vi "LAS-CTS_NDFilterScanCharge.vi"() -> ()   [LabVIEW 2024]
uses:
  <vilib>/httpClient/LabVIEWHTTPClient.lvlib
  <vilib>/Analysis/NI_AALBase.lvlib
panel:
  out "Ion Charge Chart":dbl(graph)
  out "Ion Charge (pC)":dbl format="%.3g"
  in  "Keithly":refnum<visa-resource-name>
  out "Laser Energy Chart":dbl(graph)
  out "Average Laser Energy (uJ)":dbl format="%.3g"
  out "ND Filter Position":i32
  in  "file path (use dialog)":path
  in  "# of Positions":i32
  in  "Step Size":i32
  in  "ND Filter":refnum<visa-resource-name>
  in  "Number of Pulses":i32
  out "number of measurements":i32
  out "Laser Energy (uJ)":dbl
  in  "Energy Meter":refnum<visa-resource-name>
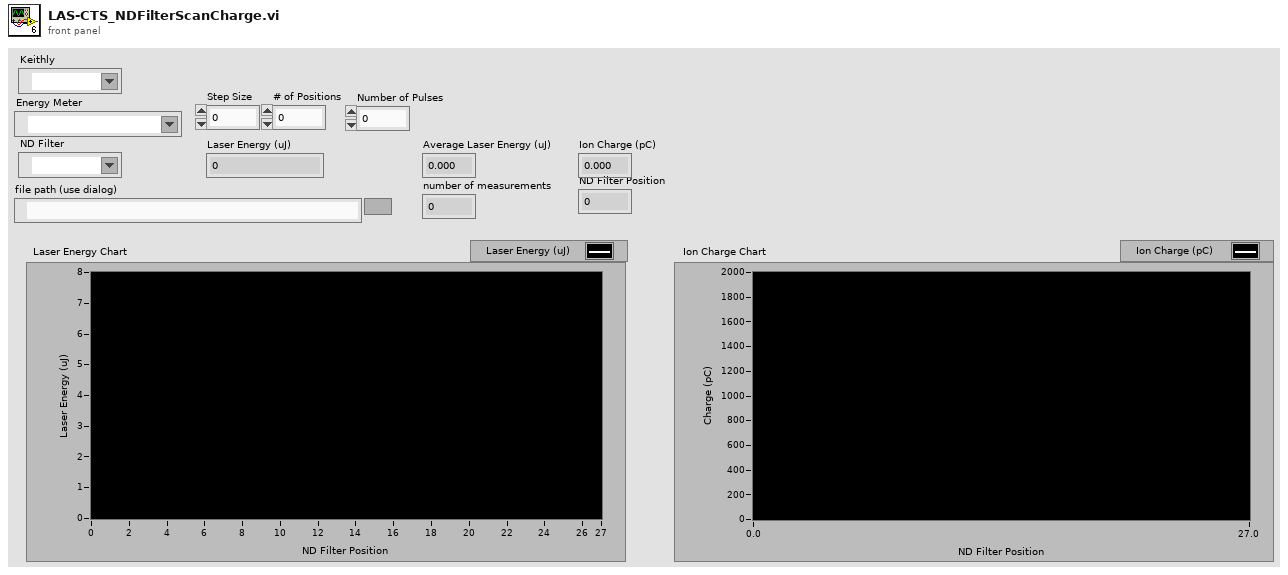
[diagram p1: front panel]
types:
  T1 = enum16{"open", "replace", "create", "open or create", "replace or create", "replace or create with confirmation"}
  T2 = typedef "LabVIEWHTTPClient.lvlib/ClientHandle.ctl" = refnum<k1>
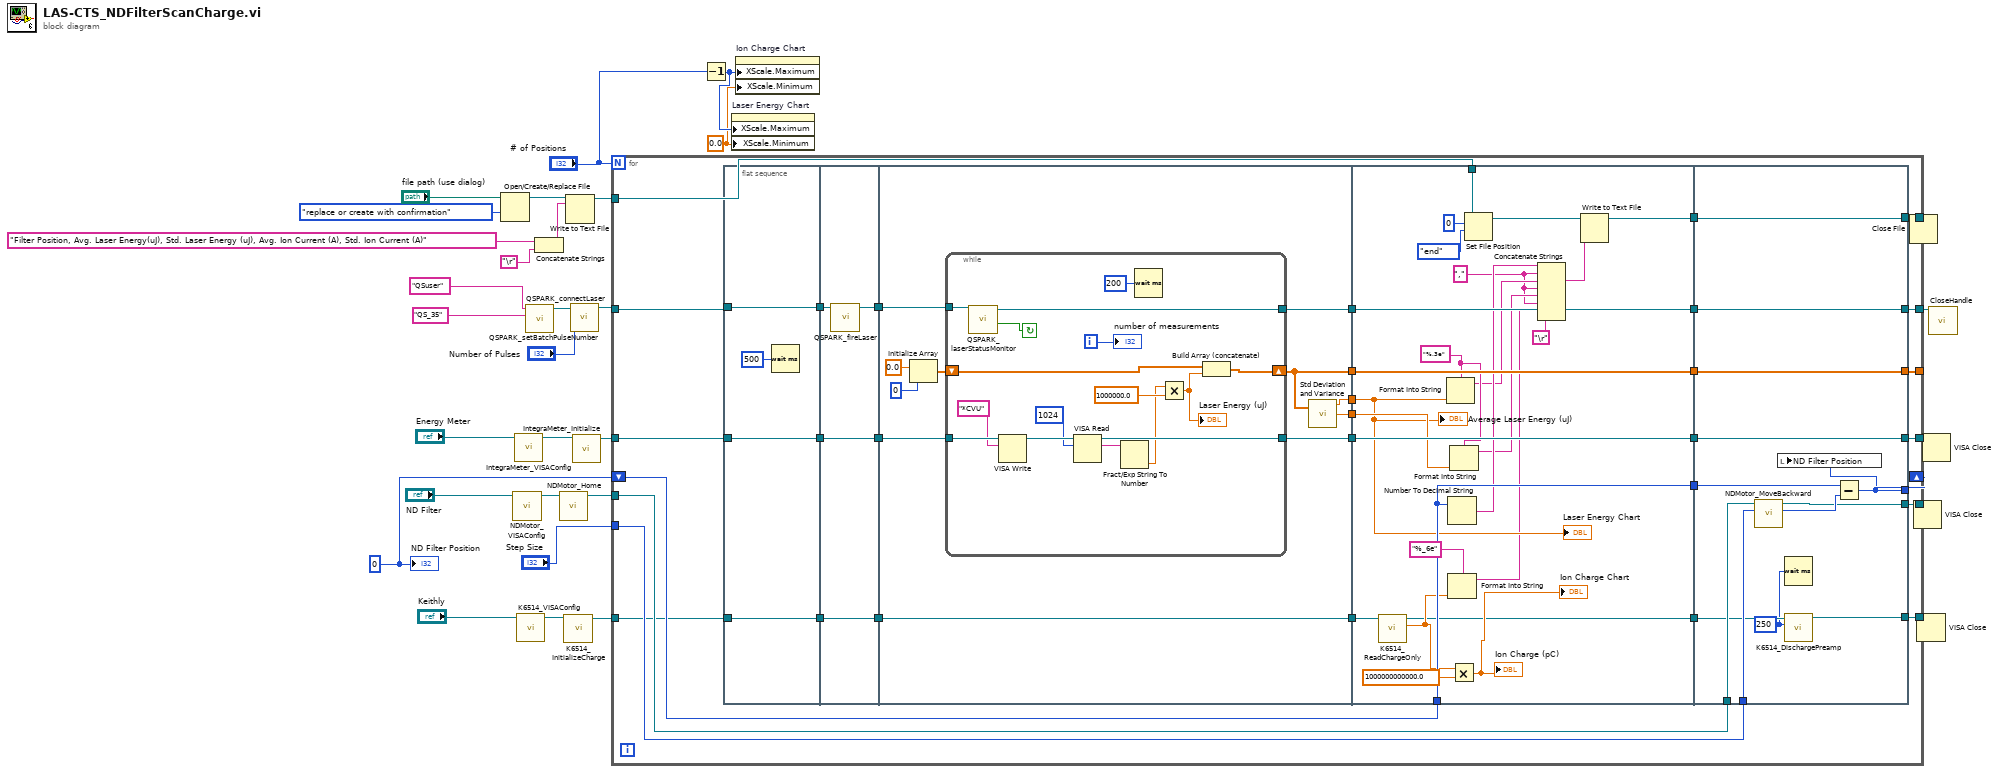
[diagram p0: block diagram]
diagram:
  w1 = 0.0 ("X Scale.Range:Minimum")
  w12 = 0 ("ND Filter Position")
  n1 = Open/Create/Replace File(file path (use dialog)="file path (use dialog)", operation (0:open)=T1."replace or create with confirmation") -> (refnum out=w11:refnum<file>)  [unwired: 4 in, 2 out]
  n2 = call "NDMotor_VISAConfig.vi"("VISA resource name"="ND Filter") -> ("reference out"=w20:refnum<visa-resource-name>)  [unwired: 9 in, 1 out]
  n3 = call "IntegraMeter_VISAConfig.vi"("VISA resource name"="Energy Meter") -> ("reference out"=w31:refnum<visa-resource-name>)  [unwired: 9 in, 1 out]
  n4 = call "K6514_VISAConfig.vi"("VISA resource name"="Keithly") -> ("reference out"=w6:refnum<visa-resource-name>)  [unwired: 9 in, 1 out]
  n5 = call "QSPARK_connectLaser.vi"("password"="QS_35", "username"="QSuser") -> ("client handle out"=w24:T2)  [unwired: 9 in]
  n6 = Concatenate Strings("Filter Position, Avg. Laser Energy(uJ), Std. Laser Energy (uJ), Avg. Ion Current (A), Std. Ion Current (A)" ("text"), "\r") -> (w15:string)
  n7 = call "NDMotor_Home.vi"("VISA resource name"=w20) -> ("VISA resource name out"=w19:refnum<visa-resource-name>)  [unwired: 9 in, 1 out]
  n8 = call "K6514_InitializeCharge.vi"("VISA resource name"=w6) -> ("VISA resource name out"=w5:refnum<visa-resource-name>)  [unwired: 9 in, 1 out]
  n9 = Write to Text File(file (use dialog)=w11, text=w15) -> (refnum out=w14:refnum<file>)  [unwired: 2 in, 2 out]
  n10 = call "QSPARK_setBatchPulseNumber.vi"("Number of Pulses"="Number of Pulses", "client handle"=w24) -> ("client handle out"=w27:T2)  [unwired: 9 in]
  n11 = call "IntegraMeter_Initialize.vi"("VISA resource name"=w31) -> ("VISA resource name out"=w29:refnum<visa-resource-name>)  [unwired: 9 in, 1 out]
  n12 = for {
    N: "# of Positions" -> [_]
    tunnel: [w57] -> _
    tunnel: "Step Size" -> [w44]
    tunnel: w14 -> [w53]
    tunnel: w27 -> [w59]
    tunnel: [w58] -> w25
    tunnel: w29 -> [w61]
    tunnel: [w60] -> w28
    tunnel: w19 -> [w42]
    tunnel: [w52] -> w13
    shift-right: [w51] -> _
    shift-left: w12 -> [w50]
    tunnel: [w43] -> w8
    tunnel: w5 -> [w38]
    tunnel: [w35] -> w4
    n13 = flat-sequence {
      tunnel: w38 -> [w65]
      tunnel: w61 -> [w66]
      tunnel: w59 -> [w67]
      tunnel: [w67] -> w34
      tunnel: [w66] -> w33
      tunnel: [w65] -> w32
      tunnel: [w71] -> w63
      tunnel: [w69] -> w62
      tunnel: [w68] -> w39
      tunnel: w34 -> [w70]
      tunnel: w33 -> [w71]
      tunnel: w32 -> [w68]
      tunnel: w63 -> [w82]
      tunnel: w62 -> [w80]
      tunnel: [w81] -> w56
      tunnel: [w79] -> w55
      tunnel: [w76] -> w54
      tunnel: [w75] -> w41
      tunnel: [w74] -> w40
      tunnel: w39 -> [w72]
      tunnel: [w72] -> w37
      tunnel: w56 -> [w123]
      tunnel: w55 -> [w122]
      tunnel: w54 -> [w121]
      tunnel: w53 -> [w118]
      tunnel: w50 -> [w114]
      tunnel: [w123] -> w49
      tunnel: [w122] -> w48
      tunnel: [w121] -> w47
      tunnel: [w116] -> w46
      tunnel: [w114] -> w45
      tunnel: w41 -> [w106]
      tunnel: w40 -> [w112]
      tunnel: w37 -> [w104]
      tunnel: [w99] -> w36
      tunnel: [w127] -> w51
      tunnel: [w133] -> w52
      tunnel: [w134] -> w57
      tunnel: [w135] -> w58
      tunnel: [w136] -> w60
      tunnel: w49 -> [w136]
      tunnel: w48 -> [w135]
      tunnel: w47 -> [w134]
      tunnel: w46 -> [w133]
      tunnel: w45 -> [w131]
      tunnel: w44 -> [w130]
      tunnel: [w129] -> w43
      tunnel: w42 -> [w128]
      tunnel: w36 -> [w126]
      tunnel: [w125] -> w35
      frame #0 {
        n14 = Wait (ms)(milliseconds to wait=u32 500) -> ()  [unwired: 1 out]
      }
      frame #1 {
        n15 = call "QSPARK_fireLaser.vi"("client handle"=w70) -> ("client handle out"=w69:T2)  [unwired: 10 in]
      }
      frame #2 {
        n16 = Initialize Array(0.0 ("element"), 0 ("dimension size")) -> (w73:dbl[])
        n17 = while {
          tunnel: w82 -> [w98]
          tunnel: [w96] -> w81
          tunnel: w80 -> [w91]
          tunnel: [w90] -> w79
          shift-right: [w87] -> w76
          shift-left: w73 -> [w88]
          i -> [w92]
          stop <- w89 continue-if-true
          n18 = call "QSPARK_laserStatusMonitor.vi"("client handle"=w91) -> ("laser on?"=w89:bool, "client handle out"=w90:T2)  [unwired: 8 in, 1 out]
          n19 = VISA Write(VISA resource name=w98, write buffer="*CVU") -> (VISA resource name out=w97:refnum<visa-resource-name>)  [unwired: 1 in, 2 out]
          n20 = VISA Read(VISA resource name=w97, byte count=u32 1024) -> (VISA resource name out=w96:refnum<visa-resource-name>, read buffer=w93:string)  [unwired: 1 in, 2 out]
          n21 = Fract/Exp String To Number(string=w93) -> (number=w84:dbl)  [unwired: 3 in, 1 out]
          n22 = Wait (ms)(milliseconds to wait=u32 200 ("millisecond multiple")) -> ()  [unwired: 1 out]
          n23 = Multiply(x=w84, y=1000000.0) -> (x*y=w83:dbl)
          "Laser Energy (uJ)" <- w83
          n24 = Build Array (concatenate)(w88, w83) -> (w87:dbl[])
          "number of measurements" <- w92
        }
        n25 = call <vilib>:"Std Deviation and Variance.vi"("X"=w76) -> ("mean"=w75:dbl, "standard deviation"=w74:dbl)  [unwired: 1 in, 1 out]
      }
      frame #3 {
        w102 = "," ("string")
        w113 = "%.3e" ("format string")
        n26 = call "K6514_ReadChargeOnly.vi"("VISA resource name"=w104) -> ("charge(C)"=w103:dbl, "VISA resource name out"=w99:refnum<visa-resource-name>)  [unwired: 6 in, 2 out]
        n27 = Format Into String(format string=w113, w106) -> (resulting string=w110:string)  [unwired: 2 in, 1 out]
        n28 = Number To Decimal String(number=w114) -> (decimal integer string=w111:string)  [unwired: 1 in]
        n29 = Format Into String(format string="%_6e", w103) -> (resulting string=w101:string)  [unwired: 2 in, 1 out]
        n30 = Format Into String(format string=w113, w112) -> (resulting string=w109:string)  [unwired: 2 in, 1 out]
        n31 = Multiply(x=w103, y=1000000000000.0) -> (x*y=→"Ion Charge (pC)" →"Ion Charge Chart":dbl)
        n32 = Set File Position(offset (in bytes) (0)=i64 0, refnum=w118, from (0:start)=enum16{"start", "end", "current"}."end") -> (refnum out=w117:refnum<file>)  [unwired: 1 in, 1 out]
        n33 = Concatenate Strings(w111, w102, w110, w102, w109, w102, w101, "\r") -> (w115:string)
        n34 = Write to Text File(file (use dialog)=w117, text=w115) -> (refnum out=w116:refnum<file>)  [unwired: 2 in, 2 out]
        "Average Laser Energy (uJ)" <- w106
        "Laser Energy Chart" <- w106
      }
      frame #4 {
        w124 = u32 250 ("discharge time (ms)")
        n35 = call "NDMotor_MoveBackward.vi"("Steps"=w130, "VISA resource name"=w128) -> ("steps"=w132:i32, "VISA resource name out"=w129:refnum<visa-resource-name>)  [unwired: 6 in, 2 out]
        n36 = Wait (ms)(milliseconds to wait=w124) -> ()  [unwired: 1 out]
        n37 = call "K6514_DischargePreamp.vi"("discharge time (ms)"=w124, "VISA resource name in"=w126) -> ("VISA resource name out"=w125:refnum<visa-resource-name>)  [unwired: 8 in, 1 out]
        n38 = Subtract(x=w131, y=w132) -> (x-y=w127:i32)
        n39 = local write "ND Filter Position"(w127) -> ()
      }
    }
  }
  n40 = Decrement(x="# of Positions") -> (x-1=w2:i32)
  n41 = property on="Laser Energy Chart" class="WFChart (strict)"("XScale.Maximum"=w2, "XScale.Minimum"=w1) -> ()  [unwired: 2 in, 2 out]
  n42 = property on="Ion Charge Chart" class="WFChart (strict)"("XScale.Maximum"=w2, "XScale.Minimum"=w1) -> ()  [unwired: 2 in, 2 out]
  n43 = Close File(refnum=w13) -> ()  [unwired: 1 in, 2 out]
  n44 = VISA Close(VISA resource name=w8) -> ()  [unwired: 1 in, 1 out]
  n45 = VISA Close(VISA resource name=w4) -> ()  [unwired: 1 in, 1 out]
  n46 = VISA Close(VISA resource name=w28) -> ()  [unwired: 1 in, 1 out]
  n47 = call <vilib>:"CloseHandle.vi"("client handle"=w25) -> ()  [unwired: 14 in, 1 out]
  "ND Filter Position" <- w12
